vi "HP 53131 Read.vi"(2 "Point #":i32, 3 "Instrument Address":refnum<visa-resource-name>) -> (0 "Stop":bool, 1 "Measurement":dbl[](array[numeric]) format="%.6e")   [LabVIEW 2020]
doc: "This VI reads a single reading from a Keithley 2001 multimeter. The stop boolean is always false. If no reading is obtained a single zero is returned.\nScott Hannahs, NHMFL-FSU, Nov 1993"
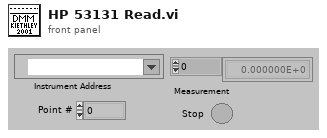
[diagram p1: front panel]
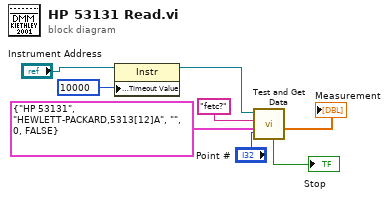
[diagram p0: block diagram]
diagram:
  n1 = property class="Instr"(reference="Instrument Address", "General Settings:Timeout Value"=u32 10000) -> (reference out=w2:refnum<visa-resource-name>)  [unwired: 1 in, 1 out]
  n2 = call "Test and Get Data.vi"("Point #"="Point #", "Instrument Info"=cluster{string, string, string, u32, bool} {"HP 53131", "HEWLETT-PACKARD,5313[12]A", "", 0, FALSE}, "Command String"="fetc?", "VISA Sesson"=w2) -> ("Measurement"=→"Measurement":dbl[], "Stop"=→"Stop":bool)  [unwired: 2 in, 3 out]
